vi "input readbacks into cluster.vi"(8 "error in (no error)":errorcluster, 9 "beamline readbacks 2":T1) -> (0 "error out":errorcluster, 1 "beamline readbacks":T1)   [LabVIEW 2016]
doc: "inputs values of beamline components into a array, which can later be used to check for problems during data collection"
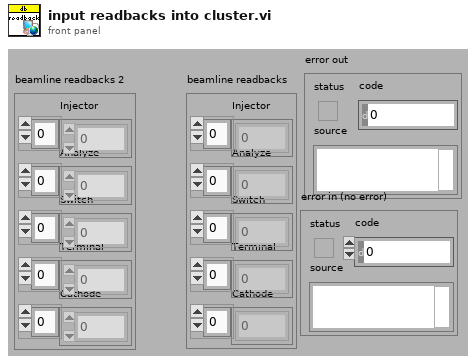
[diagram p1: front panel]
types:
  T1 = cluster{"Injector":dbl[], "Analyze":dbl[], "Switch":dbl[], "Terminal":dbl[], "Cathode":dbl[]}
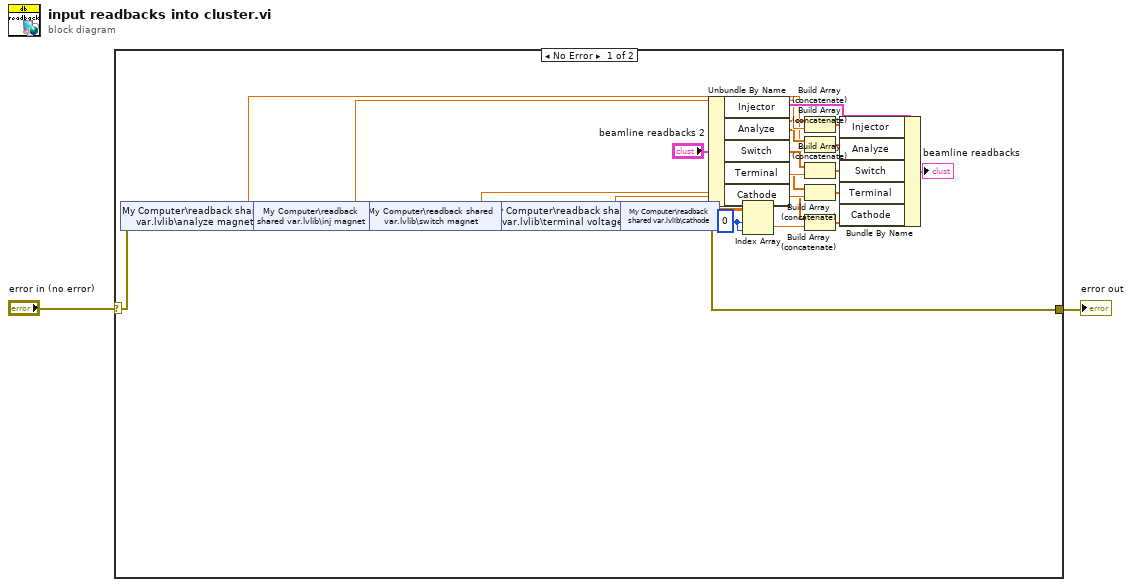
[diagram p0: block diagram]
diagram:
  n1 = case shown="No Error" "error in (no error)" {
    selector: "error in (no error)" -> [w4 w28]
    tunnel: [w3 w28] -> w2
    frame No Error {
      w26 = 0 ("disabled index (col)")
      n2 = shared-variable "My Computer\\readback shared var.lvlib\\analyze magnet"(error in=w4) -> (w20:dbl, error out=w8:errorcluster)
      n3 = shared-variable "My Computer\\readback shared var.lvlib\\inj magnet"(error in=w8) -> (w23:dbl, error out=w7:errorcluster)
      n4 = shared-variable "My Computer\\readback shared var.lvlib\\switch magnet"(error in=w7) -> (w19:dbl, error out=w6:errorcluster)
      n5 = shared-variable "My Computer\\readback shared var.lvlib\\terminal voltage"(error in=w6) -> (w16:dbl, error out=w5:errorcluster)
      n6 = shared-variable "My Computer\\readback shared var.lvlib\\cathode"(error in=w5) -> (w25:dbl[][], error out=w3:errorcluster)
      n7 = Unbundle By Name("beamline readbacks 2") -> ("Injector"=w22:dbl[], "Analyze"=w21:dbl[], "Switch"=w18:dbl[], "Terminal"=w17:dbl[], "Cathode"=w15:dbl[])
      n8 = Index Array(array=w25, index (row)=w26, index (col)=w26) -> (element=w14:dbl)
      n9 = Build Array (concatenate)(w22, w23) -> (w13:dbl[])
      n10 = Build Array (concatenate)(w21, w20) -> (w12:dbl[])
      n11 = Build Array (concatenate)(w18, w19) -> (w11:dbl[])
      n12 = Build Array (concatenate)(w17, w16) -> (w10:dbl[])
      n13 = Build Array (concatenate)(w15, w14) -> (w9:dbl[])
      n14 = Bundle By Name(cluster="beamline readbacks 2", "Injector"=w13, "Analyze"=w12, "Switch"=w11, "Terminal"=w10, "Cathode"=w9) -> (→"beamline readbacks":T1)
    }
    frame Error {
    }
  }
  "error out" <- w2
